vi "From Binary.vi"(6 "byte order":T1(ring), 8 "error in (no error)":errorcluster, 10 "Binary":string, 11 "Double Float in":refnum<class "Abs_I16 Integer.lvclass">) -> (0 "error out":errorcluster, 2 "Remaining":string, 3 "Double Float out":refnum<class "Abs_I16 Integer.lvclass">)   [LabVIEW 2021, in "Abs_I16 Integer.lvclass"]
uses:
  Abs_I16 Integer.lvclass
  Support/Type.ctl
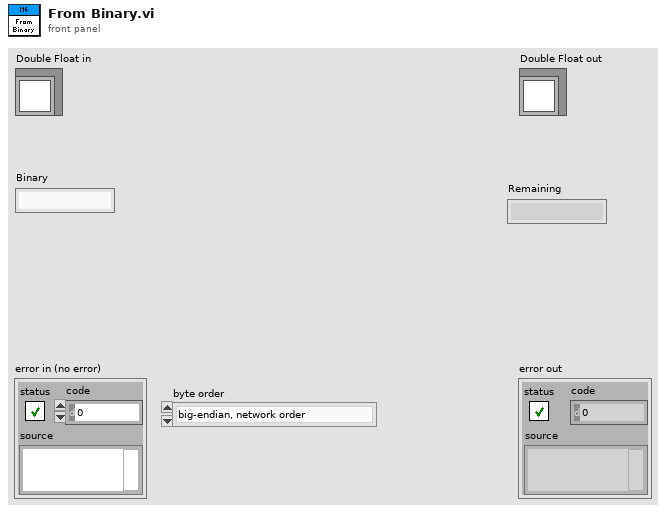
[diagram p1: front panel]
types:
  T1 = enum16{"big-endian, network order", "native, host order", "little-endian"}
  T2 = typedef "Abs_I16 Integer.lvclass/Type.ctl" = i16
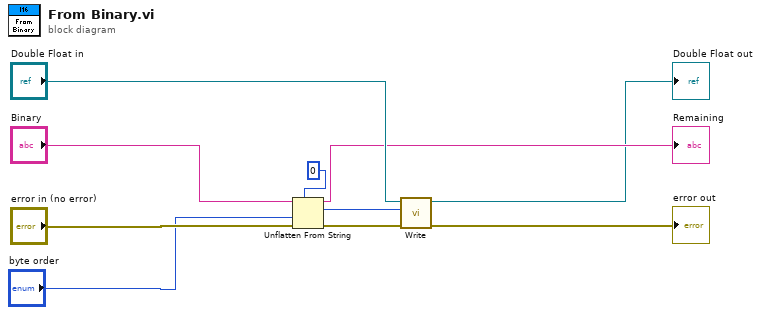
[diagram p0: block diagram]
diagram:
  n1 = Unflatten From String(type=T2 0, binary string="Binary", byte order (0:big-endian, network order)="byte order", error in (no error)="error in (no error)") -> (rest of the binary string=→"Remaining":string, value=w3:T2, error out=w2:errorcluster)  [unwired: 1 in]
  n2 = call-dynamic "Write.vi"("error in (no error)"=w2, "Value"=w3, "Double Float.lvclass_340760 in"="Double Float in") -> ("error out"=→"error out":errorcluster, "Double Float.lvclass_340760 out"=→"Double Float out":refnum<class "Abs_I16 Integer.lvclass">)  [unwired: 7 in]
